vi "restartSequence.vi"(8 "error in (no error)":errorcluster, 11 "Simon_Engine in":refnum<class "Simon_Engine.lvclass">) -> (0 "error out":errorcluster, 3 "Simon_Engine out":refnum<class "Simon_Engine.lvclass">)   [LabVIEW 2019, in "Simon_Engine.lvclass"]
doc: "Restarts the sequence for a new match."
uses:
  Simon_Engine.lvclass
  Simon_Engine.lvclass/Simon_Engine.ctl
  LED/LED Class/LED.lvclass
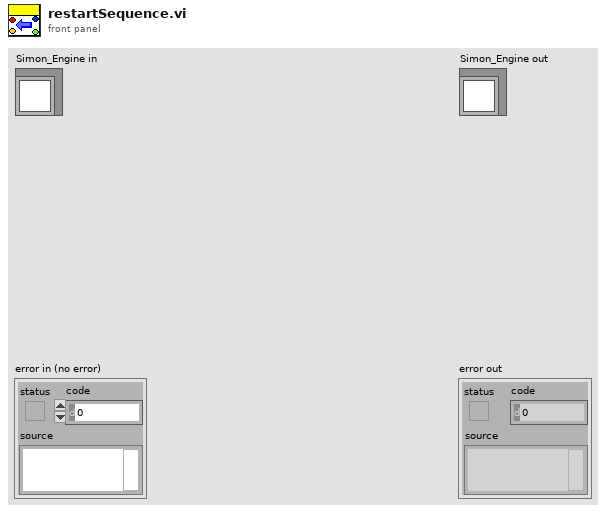
[diagram p1: front panel]
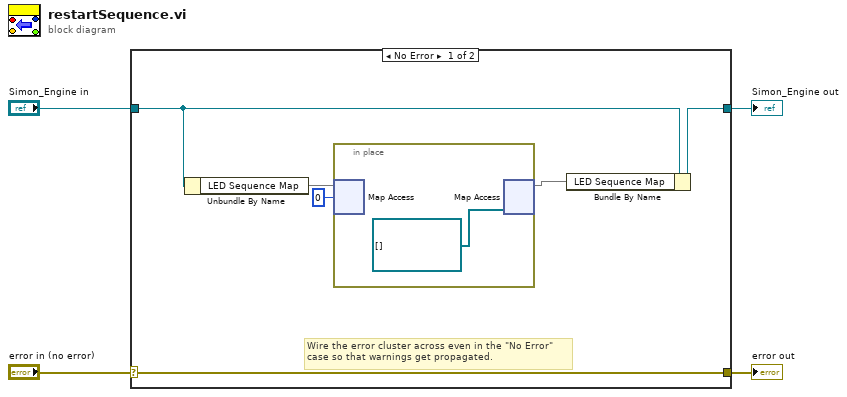
[diagram p0: block diagram]
diagram:
  n1 = case shown="No Error" "error in (no error)" {
    selector: "error in (no error)" -> [w10 w13]
    tunnel: [w10 w13] -> w3
    tunnel: [w9 w12] -> w1
    tunnel: "Simon_Engine in" -> [w8 w12]
    frame No Error {
      # "Wire the error cluster across even in the \"No Error\"\ncase so that warnings get propagated."
      n2 = Unbundle By Name(w8) -> ("LED Sequence Map"=w7:map{u8, refnum<class "LED.lvclass">[]})
      n3 = in-place {
        n4 = in-place-map #1(w7, u8 0) -> ()  [unwired: 1 in, 2 out]
        n5 = in-place-map #1(refnum<class "LED.lvclass">[] [] ("ledSequence")) -> (w5:map{u8, refnum<class "LED.lvclass">[]})  [unwired: 1 in, 2 out]
      }
      n6 = Bundle By Name(cluster=w8, "LED Sequence Map"=w5) -> (w9:refnum<class "Simon_Engine.lvclass">)
    }
    frame Error {
    }
  }
  "error out" <- w3
  "Simon_Engine out" <- w1
